vi "Flush Data Queue.vi"(8 "error in (no error)":errorcluster) -> (0 "error out":errorcluster)   [LabVIEW 2020]
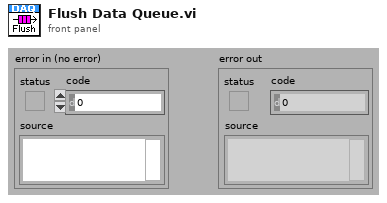
[diagram p1: front panel]
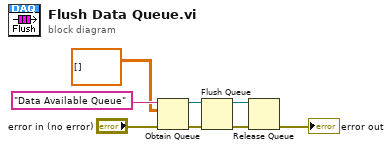
[diagram p0: block diagram]
diagram:
  n1 = Obtain Queue(name (unnamed)="Data Available Queue", element data type=dbl[][] [] ("AI Waveforms 2"), error in (no error)="error in (no error)") -> (queue out=w6:refnum<queue>, error out=w7:errorcluster)  [unwired: 2 in, 1 out]
  n2 = Flush Queue(queue=w6, error in (no error)=w7) -> (queue out=w3:refnum<queue>, error out=w4:errorcluster)  [unwired: 1 out]
  n3 = Release Queue(queue=w3, error in (no error)=w4) -> (error out=→"error out":errorcluster)  [unwired: 1 in, 2 out]
